vi "CheckParameters.vi"(8 "error in (no error)":errorcluster, 10 "Parameters":u32[](array[numeric]), 11 "Störaussendung in":refnum<class "Störaussendung.lvclass">) -> (0 "error out":errorcluster, 3 "Störaussendung out":refnum<class "Störaussendung.lvclass">)   [LabVIEW 2013, in "Störaussendung.lvclass"]
uses:
  TestInterface/TestInterface.lvclass
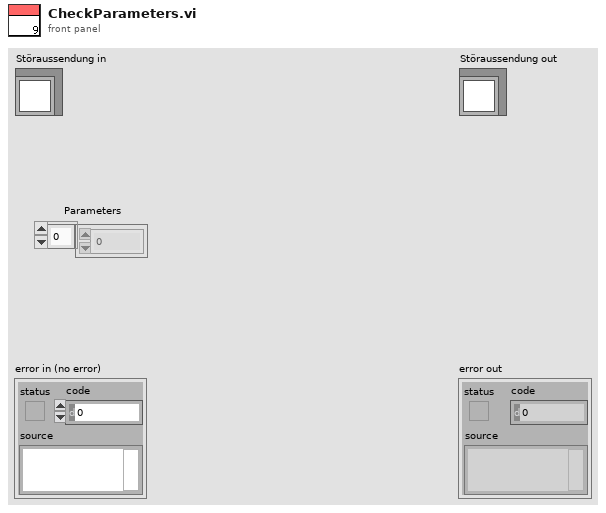
[diagram p1: front panel]
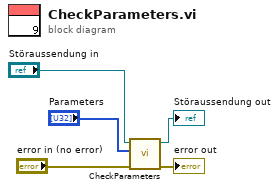
[diagram p0: block diagram]
diagram:
  n1 = call-parent "CheckParameters.vi"("error in (no error)"="error in (no error)", "Parameters"="Parameters", "TestInterface in"="Störaussendung in") -> ("error out"=→"error out":errorcluster, "TestInterface out"=→"Störaussendung out":refnum<class "Störaussendung.lvclass">)  [unwired: 7 in]
